vi "ARITHMETIC,RMS,STANDARD DEVIATION.vi"() -> ()   [LabVIEW 2015]
panel:
  out "Standard Dev":dbl
  out "RMS":dbl
  out "Arithmetic Mean":dbl
  out "initialized array 2":dbl[](array[numeric])
  in  "Numeric":dbl
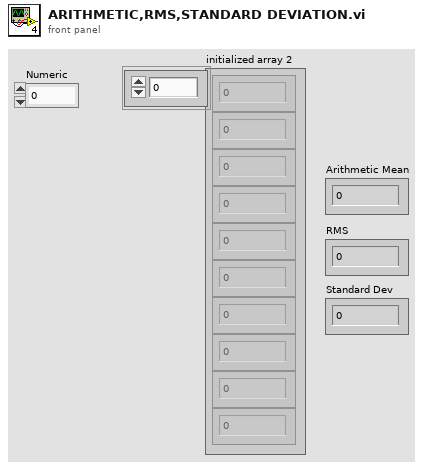
[diagram p1: front panel]
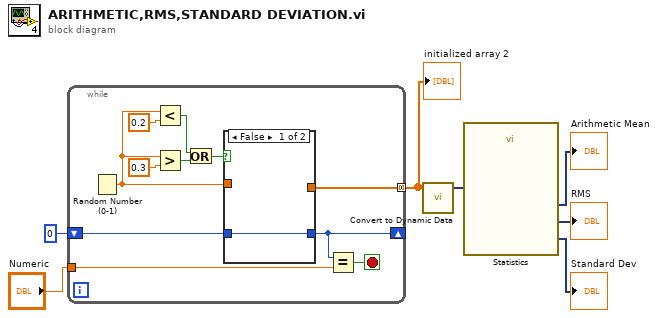
[diagram p0: block diagram]
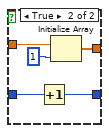
[diagram p2: hidden frame]
diagram:
  n1 = while {
    tunnel: "Numeric" -> [w17]
    tunnel: [w10] -> w6 mode=concatenating
    shift-right: [w8] -> _
    shift-left: 0 -> [w9]
    stop <- w18 stop-if-true
    n2 = Random Number (0-1)() -> (number: 0 to 1=w11:dbl)
    n3 = Less?(x=w11, y=0.2) -> (x < y?=w13:bool)
    n4 = Greater?(x=w11, y=0.3) -> (0:w14:bool)
    n5 = Or(x=w13, y=w14) -> (x .or. y?=w12:bool)
    n6 = case shown="False" w12 {
      tunnel: w11 -> [_ w24]
      tunnel: [_ w22] -> w10
      tunnel: [w19 w21] -> w8
      tunnel: w9 -> [w19 w20]
      frame False {
      }
      frame True {
        n7 = Increment(x=w20) -> (x+1=w21:i32)
        n8 = Initialize Array(w24, 1 ("dimension size")) -> (w22:dbl[])
      }
    }
    n9 = Equal?(x=w8, y=w17) -> (x = y?=w18:bool)
  }
  "initialized array 2" <- w6
  n10 = call "Convert to Dynamic Data"("Array"=w6) -> ("Dynamic Data Type"=w5:dynamicdata)  [unwired: 3 in]
  n11 = call "Statistics"("Signals"=w5) -> ("Standard Dev"=→"Standard Dev":dynamicdata, "RMS"=→"RMS":dynamicdata, "Arithmetic Mean"=→"Arithmetic Mean":dynamicdata)  [unwired: 23 in, 1 out]
